vi "Write configuration.vi"(8 "error in (no error)":errorcluster, 11 "RSA in":refnum<class "RSA.lvclass">) -> (0 "error out":errorcluster, 3 "RSA out":refnum<class "RSA.lvclass">)   [LabVIEW 2012, in "RSA.lvclass"]
doc: "Writes the configuration cluster into the configuration file. Configuration file is XML-based. It's name is <component ID>.xml"
uses:
  RSA.lvclass
  <vilib>/Distrio/Murmex/Murmex/Murmex.lvclass
  RSA.lvclass/RSA.ctl
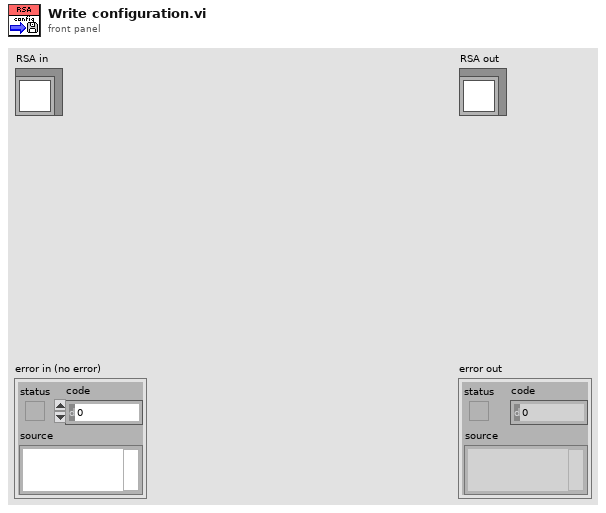
[diagram p1: front panel]
types:
  T1 = typedef "RSA.lvclass/configurationcluster.ctl" = cluster{"initialised array":dbl[]}
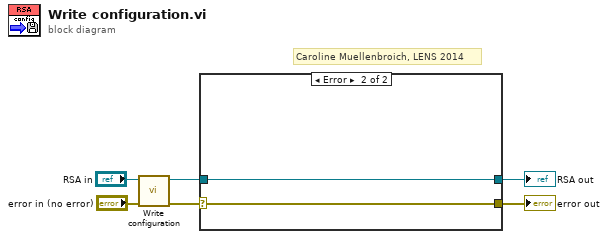
[diagram p0: block diagram]
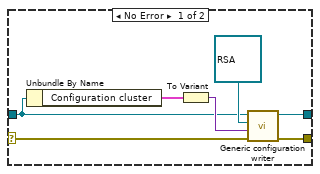
[diagram p2: hidden frame]
diagram:
  # "Caroline Muellenbroich, LENS 2014"
  n1 = call-parent "Write configuration.vi"("error in (no error)"="error in (no error)", "Murmex in"="RSA in") -> ("error out"=w4:errorcluster, "Murmex out"=w3:refnum<class "RSA.lvclass">)  [unwired: 8 in]
  n2 = case shown="Error" w4 {
    selector: w4 -> [w9 w14]
    tunnel: w3 -> [w11 w15]
    tunnel: [w8 w14] -> w2
    tunnel: [w7 w15] -> w1
    frame No Error {
      n3 = Unbundle By Name(w11) -> ("Configuration cluster"=w10:T1)
      n4 = To Variant(anything=w10) -> (Variant=w12:variant)
      n5 = call <vilib>:"Generic configuration writer.vi"("error in (no error)"=w9, "configuration"=w12, "inheritance level"=refnum<class "RSA.lvclass"> refnum ("RSA"), "MurmexBase in"=w11) -> ("error out"=w8:errorcluster, "MurmexBase out"=w7:refnum<class "RSA.lvclass">)  [unwired: 6 in]
    }
    frame Error {
    }
  }
  "error out" <- w2
  "RSA out" <- w1
